vi "ge_GetHdr.vi"(9 "error in":errorcluster, 10 "MeasType":T5, 11 "ge_DAQManDefinitions":T6) -> (1 "error out":errorcluster, 3 "Table Hdrs":T1[](array[typedef]))   [LabVIEW 2012]
uses:
  Common/Controls/DAQMan Definitions.ctl
  Custom Ctrls/ge_MeasType.ctl
  Custom Ctls Table/ge_ColDef.ctl
  Common/Controls/HeaderNames.ctl
  Custom Ctls Table/ge_HdrInfo.ctl
  Custom Ctls Table/ge_GlblCtrls.ctl
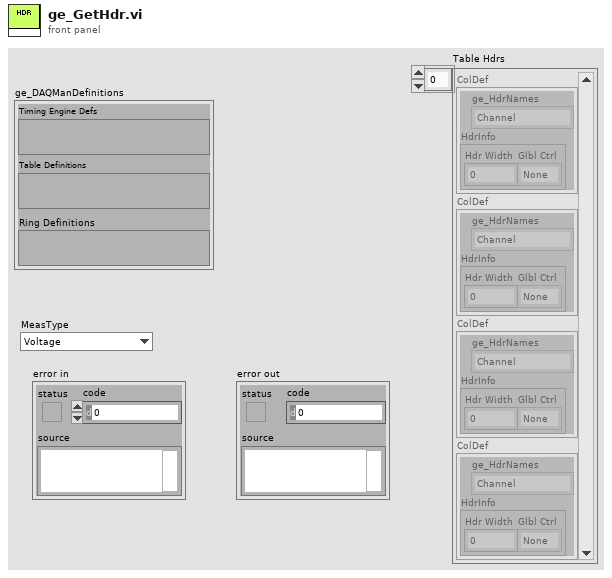
[diagram p1: front panel]
types:
  T1 = typedef "ge_ColDef.ctl" = cluster{"ge_HdrNames":T2, "HdrInfo":T3}
  T2 = typedef "HeaderNames.ctl" = enum16{"Channel", "Device", "Spacer", "Description", "MB", "Range", "Terminal", "Coupling", "Thresh (V)", "Pulse/Rev", "Slope", "Min EU", "Min RPM", "mV/EU", "Iex", "Temp Units", "Type", "CJC Src", "CJC Val", "Ro", "Wire Cfg", "Strain Mode", "Vex", "Bridge Type", "GF", "Gauge Res", "Poisson", "Lead Res", "Init Strain", "GAF", "Scale", "Offset", "Unit (EU)", "dB?", "dB Ref", "Cal Mag", "Cal Units", "Max Temp", "Min Temp", "Max Strain", "Min Strain"}
  T3 = typedef "ge_HdrInfo.ctl" = cluster{"Hdr Width":i32, "Glbl Ctrl":T4}
  T4 = typedef "ge_GlblCtrls.ctl" = enum16{"Str0", "Bool0", "Bool1", "Int0", "Ring0", "Ring1", "Ring2", "Ring3", "Dbl0", "Dbl1", "Dbl2", "Dbl3", "Cal0", "Cal1", "Cal2", "None"}
  T5 = typedef "ge_MeasType.ctl" = enum16{"Voltage", "Frequency", "Tachometer", "Dynamic", "Thermocouple", "RTD", "Strain", "Current", "Resistance"}
  T6 = typedef "DAQMan Definitions.ctl" = cluster{"Timing Engine Defs":variant, "Table Definitions":variant, "Ring Definitions":variant}
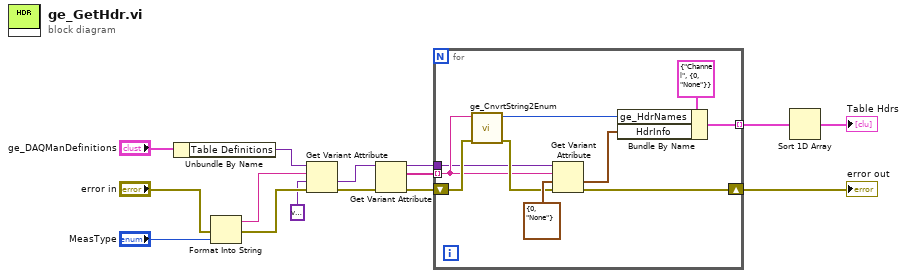
[diagram p0: block diagram]
diagram:
  n1 = Unbundle By Name("ge_DAQManDefinitions") -> ("Table Definitions"=w1:variant)
  n2 = Format Into String(error in="error in", "MeasType") -> (resulting string=w14:string, error out=w6:errorcluster)  [unwired: 2 in]
  n3 = Get Variant Attribute(Variant=w1, name=w14, default value (empty Variant)=variant ("value"), error in=w6) -> (value=w12:variant, error out=w13:errorcluster)  [unwired: 2 out]
  n4 = Get Variant Attribute(Variant=w12, error in=w13) -> (duplicate Variant=w8:variant, names=w10:string[], error out=w11:errorcluster)  [unwired: 2 in, 1 out]
  n5 = for {
    tunnel: w10 -> [w17] mode=indexing
    shift-right: [w22] -> w9
    shift-left: w11 -> [w20]
    tunnel: [w21] -> w4 mode=indexing
    tunnel: w8 -> [w16]
    n6 = call "ge_CnvrtString2Enum.vi"("error in (no error)"=w20, "Enum String"=w17) -> ("error out"=w19:errorcluster, "Hdr Name"=w18:T2)  [unwired: 8 in]
    n7 = Get Variant Attribute(Variant=w16, name=w17, default value (empty Variant)=T3 {"Hdr Width"=0, "Glbl Ctrl"=enum."None"} ("HdrInfo"), error in=w19) -> (value=w23:T3, error out=w22:errorcluster)  [unwired: 2 out]
    n8 = Bundle By Name(cluster=T1 {"ge_HdrNames"=enum."Channel", "HdrInfo"={"Hdr Width"=0, "Glbl Ctrl"=enum."None"}} ("ColDef"), "ge_HdrNames"=w18, "HdrInfo"=w23) -> (w21:T1)
  }
  "error out" <- w9
  n9 = Sort 1D Array(array=w4) -> (sorted array=→"Table Hdrs":T1[])
